vi "Bias Spec.vi"(7 "Scan Parameters in":T1 {"Avoid zero threshold (V)" format="%#_13g"}, 8 "error in (no error)":errorcluster, 9 "Cluster":cluster{"Initial x":dbl, "Initial y":dbl}, 10 "ScanQ in":refnum<queue>, 11 "Queue in":refnum<queue>) -> (0 "error out":errorcluster, 1 "output cluster":cluster{"Initial x":dbl, "Initial y":dbl}, 2 "ScanQ out":refnum<queue>, 3 "Queue out":refnum<queue>, 5 "Scan Parameters out":T1 {"Avoid zero threshold (V)" format="%#_13g"})   [LabVIEW 2025]
uses:
  CTLS/ACK.ctl
  <userlib>/Nanonis Prog Interface V5e/Nanonis Prog Interface.lvlib
  CTLS/Scan_Params (QMH).ctl
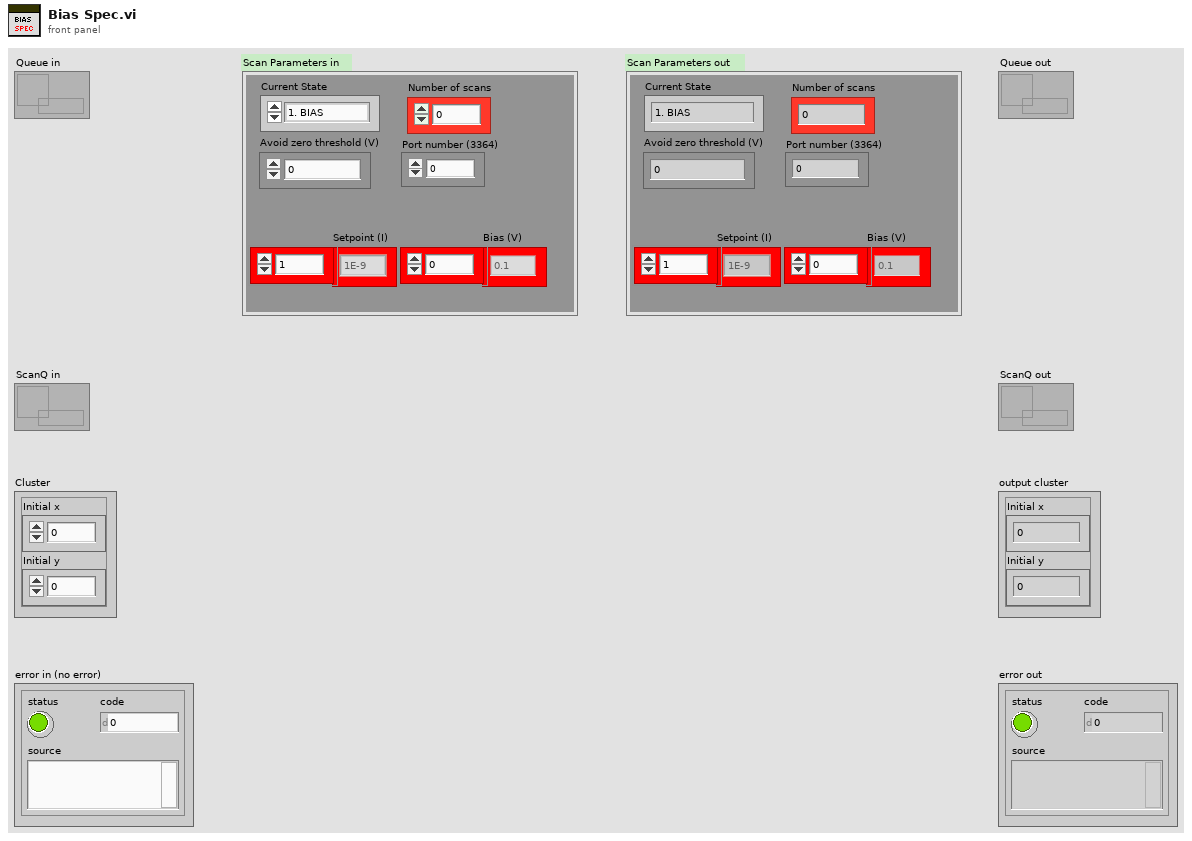
[diagram p1: front panel]
types:
  T1 = typedef "Scan_Params (QMH).ctl" = cluster{"Setpoint (I)":dbl[], "Bias (V)":dbl[], "Number of scans":u8, "Port number (3364)":u32, "Avoid zero threshold (V)":dbl, "Current State":enum16{"1. BIAS", "2. POLL BIAS", "3. SCAN", "4. SCAN_IDLE", "5. Drift_Correct (SF)", "6. Drift_Correct (BS)", "7. STOP"}}
  T2 = enum16{"1. None", "2. TempStable", "3. FieldStable", "4. ConfigApplied", "5. ScanDone", "6. BiasDone", "7. DriftDone (SF)", "8. DrifDone (BS)"}
  T3 = typedef "ACK.ctl" = cluster{"ACK":enum16{"1. None", "2. TempStable", "3. FieldStable", "4. ConfigApplied", "5. ScanDone", "6. BiasDone", "7. DriftDone (SF)", "8. DrifDone (BS)"}}
  T4 = enum16{"1. BIAS", "2. POLL BIAS", "3. SCAN", "4. SCAN_IDLE", "5. Drift_Correct (SF)", "6. Drift_Correct (BS)", "7. STOP"}
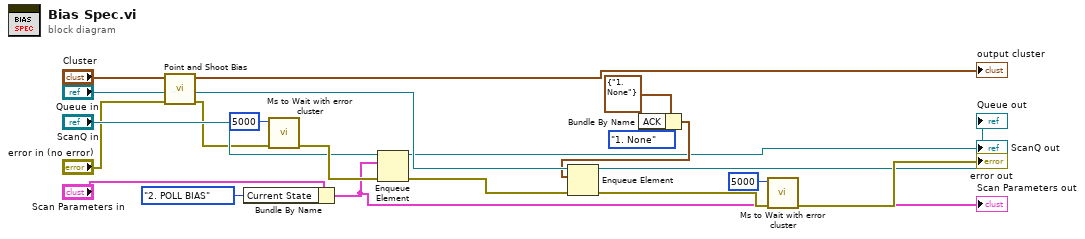
[diagram p0: block diagram]
diagram:
  n1 = call "Point and Shoot Bias.vi"("Error in (no error)"="error in (no error)", "Cluster"="Cluster") -> ("error out"=w2:errorcluster, "output cluster"=→"output cluster":cluster{"Initial x":dbl, "Initial y":dbl})  [unwired: 8 in]
  n2 = Bundle By Name(cluster="Scan Parameters in", "Current State"=T4."2. POLL BIAS") -> (w8:T1)
  "Scan Parameters out" <- w8
  n3 = call <userlib>:"Ms to Wait with error cluster.vi"("error in (no error)"=w2, "milliseconds to wait"=u32 5000) -> ("error out"=w20:errorcluster)  [unwired: 4 in, 1 out]
  n4 = Enqueue Element(queue="ScanQ in", element=w8, error in (no error)=w20) -> (queue out=→"ScanQ out":refnum<queue>, error out=w13:errorcluster)  [unwired: 1 in, 1 out]
  n5 = Bundle By Name(cluster=T3 {"ACK"=enum."1. None"} ("Acknowledements"), "ACK"=T2."1. None") -> (w9:T3)
  n6 = Enqueue Element(queue="Queue in", element=w9, error in (no error)=w13) -> (queue out=→"Queue out":refnum<queue>, error out=w15:errorcluster)  [unwired: 1 in, 1 out]
  n7 = call <userlib>:"Ms to Wait with error cluster.vi"("error in (no error)"=w15, "milliseconds to wait"=u32 5000) -> ("error out"=→"error out":errorcluster)  [unwired: 4 in, 1 out]
